vi "Open Waveform File.vi"(4 "Data Type":T1(ring)=enum."float32", 6 "File Type ID":string="WFM", 8 "Error In":errorcluster, 9 "WFM Block":waveform(dbl)[](array[waveform]), 10 "Block Interval":dbl, 11 "File Path":path) -> (0 "Error Out":errorcluster, 3 "File Refnum Out":refnum<file>)   [LabVIEW 2015]
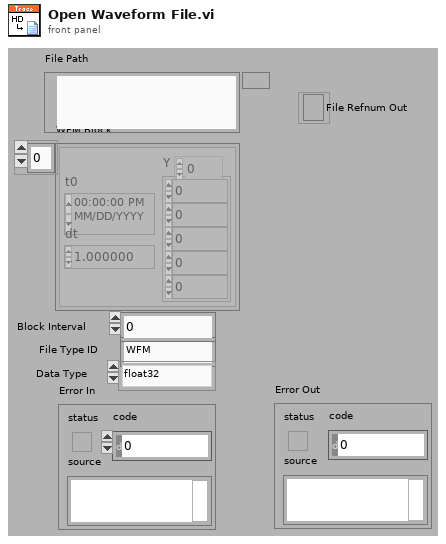
[diagram p1: front panel]
types:
  T1 = enum16{"int8", "int16", "int32", "uint8", "uint16", "uint32", "float32", "float64"}
  T2 = enum16{"open", "replace", "create", "open or create", "replace or create", "replace or create with confirmation"}
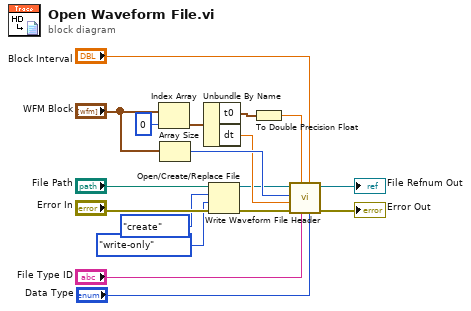
[diagram p0: block diagram]
diagram:
  n1 = Index Array(array="WFM Block", index=0) -> (element=w14:waveform(dbl))
  n2 = Array Size(array="WFM Block") -> (size(s)=w10:i32)
  n3 = Unbundle By Name(w14) -> ("t0"=w13:timestamp, "dt"=w7:dbl)
  n4 = Open/Create/Replace File(file path (use dialog)="File Path", error in="Error In", operation (0:open)=T2."create", access (0:read/write)=enum16{"read/write", "read-only", "write-only"}."write-only") -> (refnum out=w6:refnum<file>, error out=w4:errorcluster)  [unwired: 2 in, 1 out]
  n5 = To Double Precision Float(number=w13) -> (double precision float=w9:dbl)
  n6 = call "Write Waveform File Header.vi"("Data Type"="Data Type", "Block Interval"="Block Interval", "File Type ID"="File Type ID", "Start Time"=w9, "Error In"=w4, "Sample Interval"=w7, "No. of Channels"=w10, "File Refnum In"=w6) -> ("Error Out"=→"Error Out":errorcluster, "File Refnum Out"=→"File Refnum Out":refnum<file>)  [unwired: 2 in]
